vi "PosFileCheck.vi"(6 "Iteration":i32, 8 "MC active?":bool, 10 "UUID":string, 11 "Contacts":T1[](array[typedef])) -> (1 "File empty?":bool, 2 "Delete":bool)   [LabVIEW 2014]
uses:
  Libraries/Contact Data/Contact.ctl
  Libraries/Contact Data/Position.ctl
  Libraries/Contact Data/Controls.ctl
  Libraries/Contact Data/DestinationCluster.ctl
  Libraries/Contact Data/DesinationControls.ctl
  Libraries/Contact Data/PathData.ctl
  PathFinder/Controls/ShortestPath.ctl
  Libraries/Contact Data/Contact Data.lvlib
panel:
  out "Array":cluster{"UUID":string, "Int":i32}[](array[cluster])
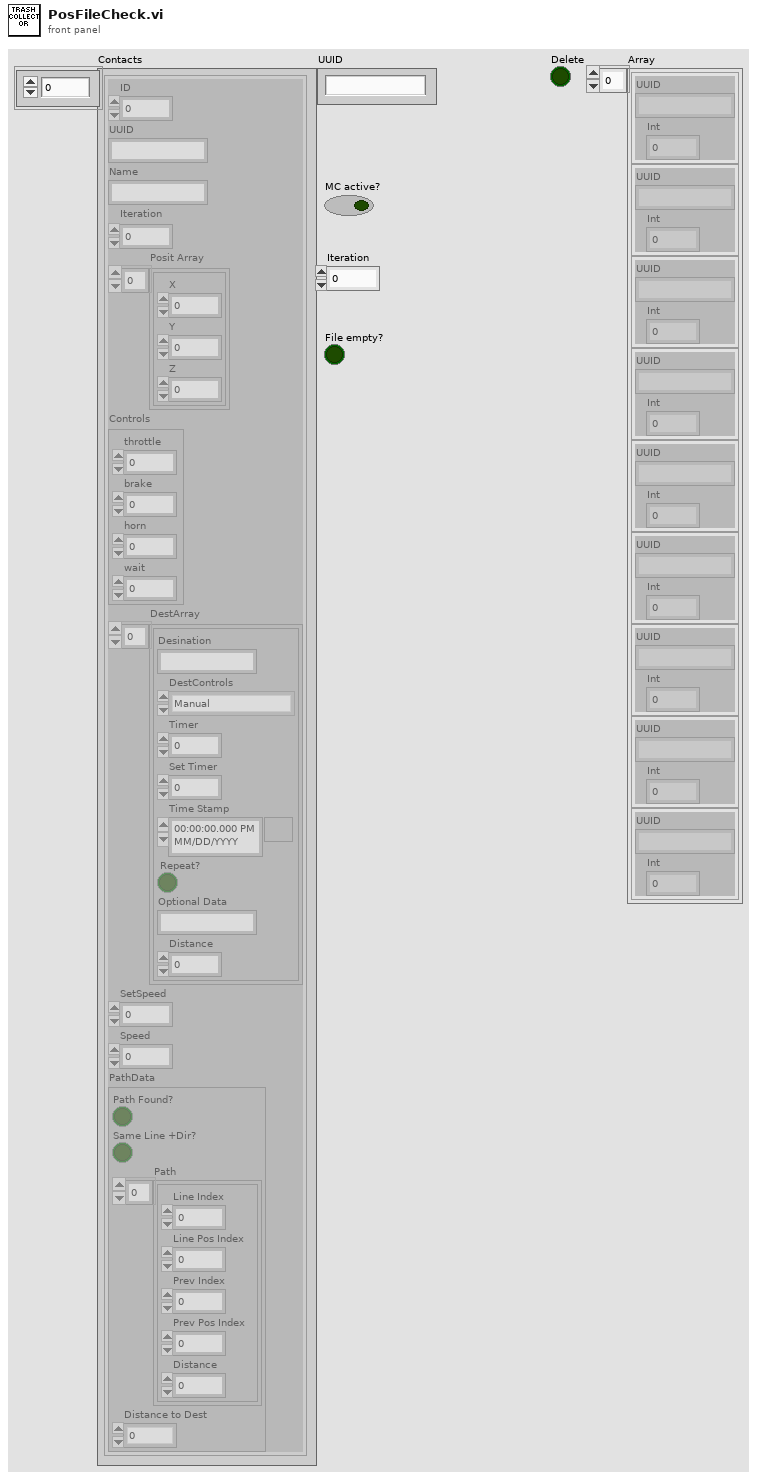
[diagram p1: front panel]
types:
  T1 = typedef "Contact Data.lvlib/Contact.ctl" = cluster{"ID":u32, "UUID":string, "Name":string, "Iteration":i32, "Posit Array":T2[], "Controls":T3, "DestArray":T4[], "SetSpeed":dbl, "Speed":dbl, "PathData":T6}
  T2 = typedef "Contact Data.lvlib/Position.ctl" = cluster{"X":dbl, "Y":dbl, "Z":dbl}
  T3 = typedef "Contact Data.lvlib/Controls.ctl" = cluster{"throttle":dbl, "brake":dbl, "horn":dbl, "wait":dbl}
  T4 = typedef "Contact Data.lvlib/DestinationCluster.ctl" = cluster{"Desination":string, "DestControls":T5, "Timer":u32, "Set Timer":u32, "Time Stamp":timestamp, "Repeat?":bool, "Optional Data":string, "Distance":dbl}
  T5 = typedef "Contact Data.lvlib/DesinationControls.ctl" = enum16{"Tracker", "Manual", "Stop", "Station DateTime", "Station Timer", "Maintain"}
  T6 = typedef "Contact Data.lvlib/PathData.ctl" = cluster{"Path Found?":bool, "Same Line +Dir?":bool, "Path":T7[], "Distance to Dest":dbl}
  T7 = typedef "ShortestPath.ctl" = cluster{"Line Index":i32, "Line Pos Index ":i32, "Prev Index ":i32, "Prev Pos Index":i32, "Distance":dbl}
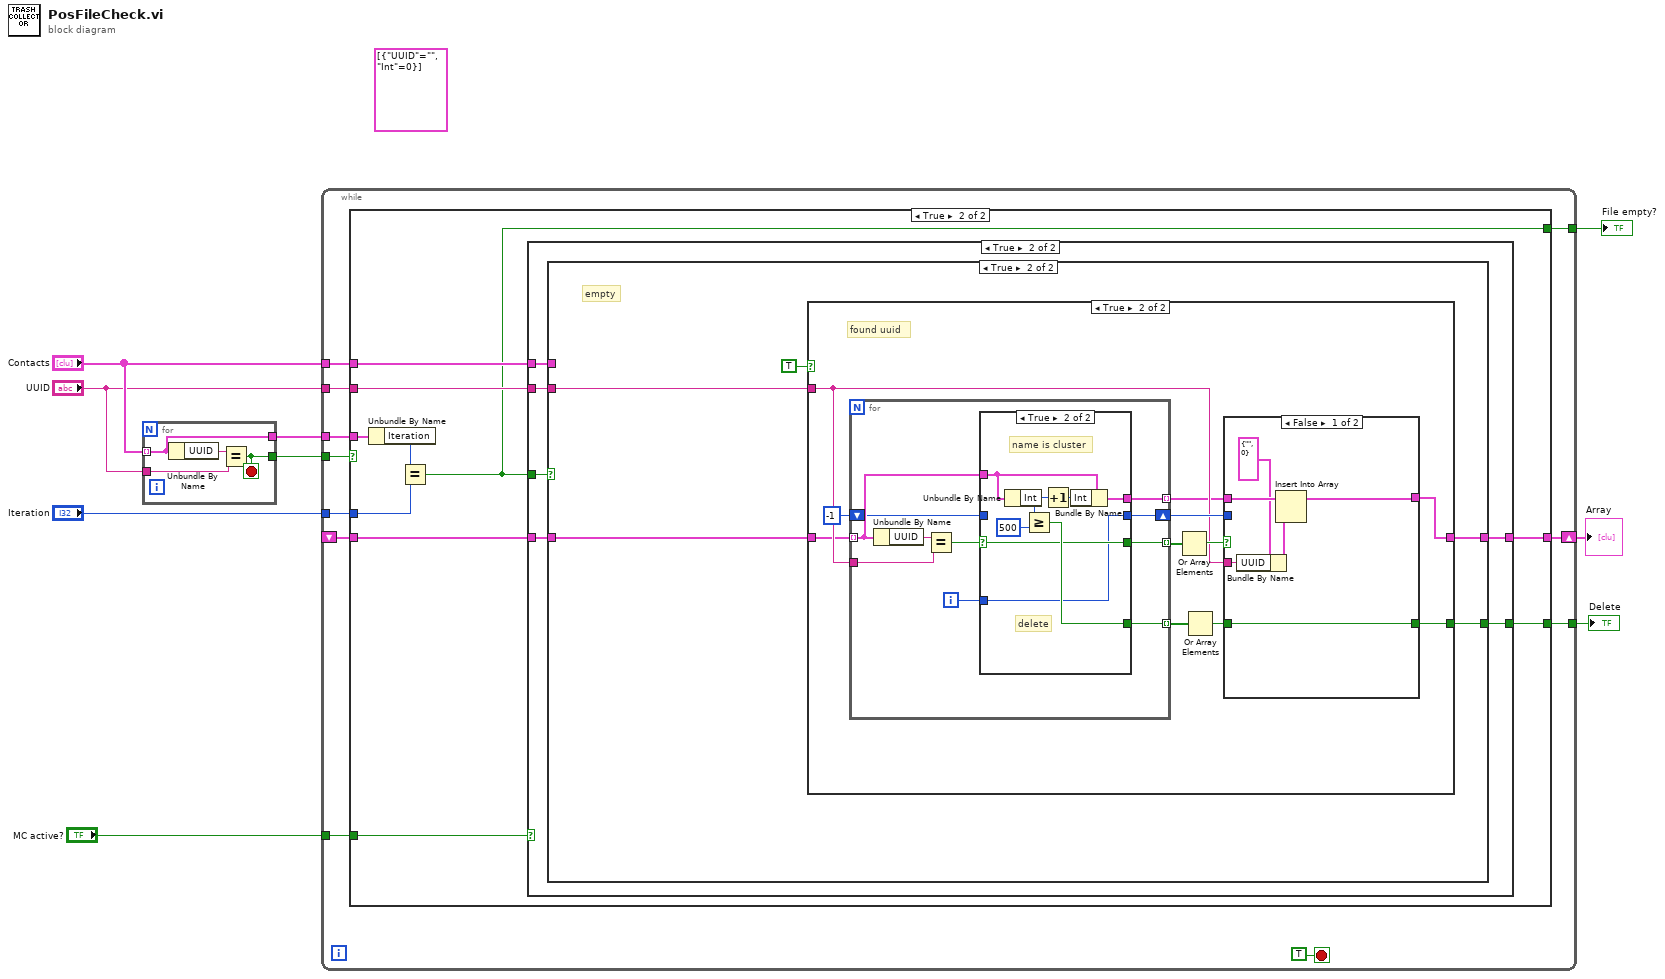
[diagram p0: block diagram]
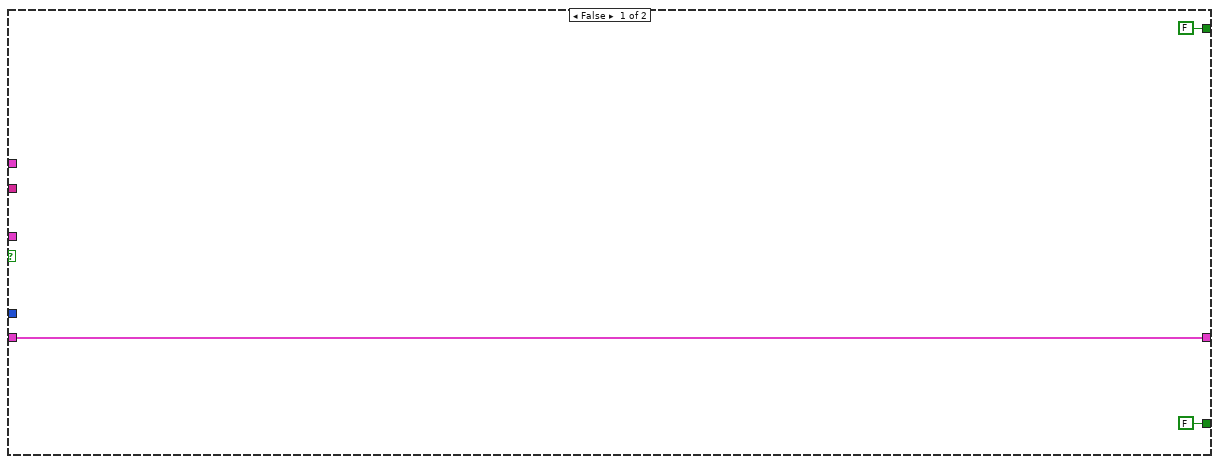
[diagram p2: hidden frame]
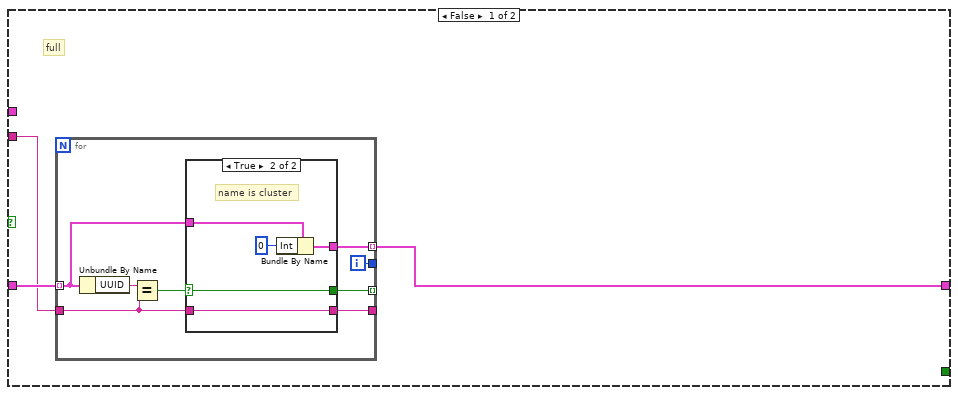
[diagram p4: hidden frame]
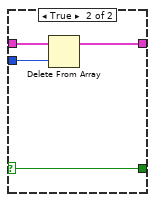
[diagram p8: hidden frame]
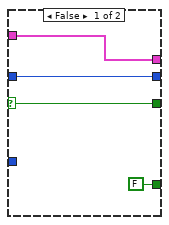
[diagram p9: hidden frame]
diagram:
  (unwired) cluster{"UUID":string, "Int":i32}[] [{"UUID"="", "Int"=0}]
  n1 = for {
    tunnel: "UUID" -> [w12]
    tunnel: "Contacts" -> [w11] mode=indexing
    tunnel: [w11] -> w4
    tunnel: [w10] -> w2
    stop <- w10 stop-if-true
    n2 = Unbundle By Name(w11) -> ("UUID"=w13:string)
    n3 = Equal?(x=w13, y=w12) -> (x = y?=w10:bool)
  }
  n4 = while {
    tunnel: "Contacts" -> [w24]
    tunnel: "UUID" -> [w23]
    shift-right: [w21] -> w8
    shift-left: _ -> [w22]
    tunnel: [w20] -> w9
    tunnel: "MC active?" -> [w19]
    tunnel: w4 -> [w18]
    tunnel: "Iteration" -> [w17]
    tunnel: w2 -> [w14]
    tunnel: [w16] -> w1
    stop <- TRUE stop-if-true
    n5 = case shown="True" w14 {
      tunnel: w24 -> [_ w37]
      tunnel: w23 -> [_ w36]
      tunnel: w22 -> [w25 w35]
      tunnel: [w25 w34] -> w21
      tunnel: [FALSE w33] -> w20
      tunnel: w19 -> [_ w32]
      tunnel: w18 -> [_ w30]
      tunnel: w17 -> [_ w29]
      tunnel: [FALSE w28] -> w16
      frame False {
      }
      frame True {
        n6 = Unbundle By Name(w30) -> ("Iteration"=w31:i32)
        n7 = Equal?(x=w31, y=w29) -> (x = y?=w28:bool)
        n8 = case shown="True" w32 {
          tunnel: w37 -> [_ w44]
          tunnel: w36 -> [_ w43]
          tunnel: w35 -> [w38 w42]
          tunnel: [w38 w41] -> w34
          tunnel: [_ w40] -> w33
          tunnel: w28 -> [_ w39]
          frame False {
          }
          frame True {
            n9 = case shown="True" w39 {
              tunnel: w44 -> [_ _]
              tunnel: w43 -> [w45 w65]
              tunnel: w42 -> [w47 w68]
              tunnel: [w46 w67] -> w41
              tunnel: [_ w66] -> w40
              frame False {
                # "full"
                n10 = for {
                  tunnel: w45 -> [w51]
                  tunnel: w47 -> [w55] mode=indexing
                  tunnel: [w53] -> _ mode=indexing
                  tunnel: [w52] -> w46 mode=indexing
                  tunnel: [w50] -> _
                  tunnel: [w49] -> _
                  i -> [w49]
                  n11 = Unbundle By Name(w55) -> ("UUID"=w54:string)
                  n12 = Equal?(x=w54, y=w51) -> (x = y?=w48:bool)
                  n13 = case shown="True" w48 {
                    selector: w48 -> [w57 w60]
                    tunnel: w55 -> [w58 w63]
                    tunnel: [w58 w62] -> w52
                    tunnel: [w57 w60] -> w53
                    tunnel: [w56 w61] -> w50
                    tunnel: w51 -> [w56 w61]
                    frame False {
                    }
                    frame True {
                      # "name is cluster"
                      n14 = Bundle By Name(cluster=w63, "Int"=0) -> (w62:cluster{"UUID":string, "Int":i32})
                    }
                  }
                }
              }
              frame True {
                # "empty"
                n15 = case shown="True" TRUE {
                  tunnel: w65 -> [_ w73]
                  tunnel: w68 -> [w69 w72]
                  tunnel: [w69 w75] -> w67
                  tunnel: [_ w74] -> w66
                  frame False {
                    # "no uuid"
                  }
                  frame True {
                    # "found uuid"
                    n16 = for {
                      tunnel: w73 -> [w104]
                      tunnel: w72 -> [w107] mode=indexing
                      tunnel: [w105] -> w80 mode=indexing
                      tunnel: [w103] -> w78 mode=indexing
                      tunnel: [w101] -> w71 mode=indexing
                      shift-right: [w99] -> w76
                      shift-left: -1 -> [w98]
                      i -> [w100]
                      n17 = Unbundle By Name(w107) -> ("UUID"=w106:string)
                      n18 = Equal?(x=w106, y=w104) -> (x = y?=w102:bool)
                      n19 = case shown="True" w102 {
                        selector: w102 -> [w110 w113]
                        tunnel: w107 -> [w111 w119]
                        tunnel: [w111 w118] -> w101
                        tunnel: [w110 w113] -> w105
                        tunnel: [FALSE w114] -> w103
                        tunnel: w100 -> [_ w112]
                        tunnel: [w109 w112] -> w99
                        tunnel: w98 -> [w109 _]
                        frame False {
                        }
                        frame True {
                          # "name is cluster"
                          # "delete"
                          n20 = Unbundle By Name(w119) -> ("Int"=w117:i32)
                          n21 = Greater Or Equal?(x=w117, y=500) -> (x >= y?=w114:bool)
                          n22 = Increment(x=w117) -> (x+1=w115:i32)
                          n23 = Bundle By Name(cluster=w119, "Int"=w115) -> (w118:cluster{"UUID":string, "Int":i32})
                        }
                      }
                    }
                    n24 = Or Array Elements(Boolean array=w80) -> (logical OR=w79:bool)
                    n25 = Or Array Elements(Boolean array=w78) -> (logical OR=w77:bool)
                    n26 = case shown="False" w79 {
                      tunnel: w71 -> [w86 w90]
                      tunnel: w73 -> [w83 _]
                      tunnel: [w82 w88] -> w75
                      tunnel: w77 -> [w81 w91]
                      tunnel: [w81 w89] -> w74
                      tunnel: w76 -> [_ w87]
                      frame False {
                        n27 = Bundle By Name(cluster=cluster{"UUID":string, "Int":i32} {"UUID"="", "Int"=0} ("new element/subarray"), "UUID"=w83) -> (w84:cluster{"UUID":string, "Int":i32})
                        n28 = Insert Into Array(array=w86, new element=w84) -> (w82:cluster{"UUID":string, "Int":i32}[])  [unwired: 1 in]
                      }
                      frame True {
                        n29 = case shown="False" w91 {
                          selector: w91 -> [w92 w97]
                          tunnel: w90 -> [w93 w96]
                          tunnel: [w92 w97] -> w89
                          tunnel: [w93 w95] -> w88
                          tunnel: w87 -> [_ w94]
                          frame False {
                          }
                          frame True {
                            n30 = Delete From Array(array=w96, index=w94) -> (array with subset deleted=w95:cluster{"UUID":string, "Int":i32}[])  [unwired: 1 in, 1 out]
                          }
                        }
                      }
                    }
                  }
                }
              }
            }
          }
        }
      }
    }
  }
  "Delete" <- w9
  "Array" <- w8
  "File empty?" <- w1
